vi "Scan and Trace.vi"() -> ()   [LabVIEW 2020]
uses:
  Global Parameters.vi
  <vilib>/Utility/file.llb/Write Delimited Spreadsheet (DBL).vi
panel:
  out "x-y":u32
  out "Laser On":bool
  in  "set trace data save rate(ms)":u32
  out "Current Position":dbl[](array[numeric])
  in  "stop":bool
  in  "Tab Control":T1(tab)
  in  "Graph path":path=path "I:/scan map test"
  out "Intensity Graph":dbl[][](graph)=[[150150.0, 0.0, 0.0, 0.0, 0.0, 0.0, 0.0, 0.0, 0.0, 0.0, 0.0, 0.0, 0.0, 0.0, 0.0, 0.0, 0.0, 0.0, 0.0, 0.0, 0.0, 0.0, 0.0, 0.0, 0.0, 0.0, 0.0, 0.0, 0.0, 0.0, 0.0], [150150.0, 0.0, 0.0, 0.0, 0.0, 0.0, 0.0, 0.0, 0.0, 0.0, 0.0, 0.0, 0.0, 0.0, 0.0, 0.0, 0.0, 0.0, 0.0, 0.0, 0.0, 0.0, 0.0, 0.0, 0.0, 0.0, 0.0, 0.0, 0.0, 0.0, 0.0], [150150.0, 0.0, 0.0, 0.0, 0.0, 0.0, 0.0, 0.0, 0.0, 0.0, 0.0, 0.0, 0.0, 0.0, 0.0, 0.0, 0.0, 0.0, 0.0, 0.0, 0.0, 0.0, 0.0, 0.0, 0.0, 0.0, 0.0, 0.0, 0.0, 0.0, 0.0], [150150.0, 0.0, 0.0, 0.0, 0.0, 0.0, 0.0, 0.0, 0.0, 0.0, 0.0, 0.0, 0.0, 0.0, 0.0, 0.0, 0.0, 0.0, 0.0, 0.0, 0.0, 0.0, 0.0, 0.0, 0.0, 0.0, 0.0, 0.0, 0.0, 0.0, 0.0], [150150.0, 0.0, 0.0, 0.0, 0.0, 0.0, 0.0, 0.0, 0.0, 0.0, 0.0, 0.0, 0.0, 0.0, 0.0, 0.0, 0.0, 0.0, 0.0, 0.0, 0.0, 0.0, 0.0, 0.0, 0.0, 0.0, 0.0, 0.0, 0.0, 0.0, 0.0], [150150.0, 0.0, 0.0, 0.0, 0.0, 0.0, 0.0, 0.0, 0.0, 0.0, 0.0, 0.0, 0.0, 0.0, 0.0, 0.0, 0.0, 0.0, 0.0, 0.0, 0.0, 0.0, 0.0, 0.0, 0.0, 0.0, 0.0, 0.0, 0.0, 0.0, 0.0], [150150.0, 0.0, 0.0, 0.0, 0.0, 0.0, 0.0, 0.0, 0.0, 0.0, 0.0, 0.0, 0.0, 0.0, 0.0, 0.0, 0.0, 0.0, 0.0, 0.0, 0.0, 0.0, 0.0, 0.0, 0.0, 0.0, 0.0, 0.0, 0.0, 0.0, 0.0], [150150.0, 0.0, 0.0, 0.0, 0.0, 0.0, 0.0, 0.0, 0.0, 0.0, 0.0, 0.0, 0.0, 0.0, 0.0, 0.0, 0.0, 0.0, 0.0, 0.0, 0.0, 0.0, 0.0, 0.0, 0.0, 0.0, 0.0, 0.0, 0.0, 0.0, 0.0], [150150.0, 0.0, 0.0, 0.0, 0.0, 0.0, 0.0, 0.0, 0.0, 0.0, 0.0, 0.0, 0.0, 0.0, 0.0, 0.0, 0.0, 0.0, 0.0, 0.0, 0.0, 0.0, 0.0, 0.0, 0.0, 0.0, 0.0, 0.0, 0.0, 0.0, 0.0], [150150.0, 0.0, 0.0, 0.0, 0.0, 0.0, 0.0, 0.0, 0.0, 0.0, 0.0, 0.0, 0.0, 0.0, 0.0, 0.0, 0.0, 0.0, 0.0, 0.0, 0.0, 0.0, 0.0, 0.0, 0.0, 0.0, 0.0, 0.0, 0.0, 0.0, 0.0], [150150.0, 0.0, 0.0, 0.0, 0.0, 0.0, 0.0, 0.0, 0.0, 0.0, 0.0, 0.0, 0.0, 0.0, 0.0, 0.0, 0.0, 0.0, 0.0, 0.0, 0.0, 0.0, 0.0, 0.0, 0.0, 0.0, 0.0, 0.0, 0.0, 0.0, 0.0], [150150.0, 0.0, 0.0, 0.0, 0.0, 0.0, 0.0, 0.0, 0.0, 0.0, 0.0, 0.0, 0.0, 0.0, 0.0, 0.0, 0.0, 0.0, 0.0, 0.0, 0.0, 0.0, 0.0, 0.0, 0.0, 0.0, 0.0, 0.0, 0.0, 0.0, 0.0], [150150.0, 0.0, 0.0, 0.0, 0.0, 0.0, 0.0, 0.0, 0.0, 0.0, 0.0, 0.0, 0.0, 0.0, 0.0, 0.0, 0.0, 0.0, 0.0, 0.0, 0.0, 0.0, 0.0, 0.0, 0.0, 0.0, 0.0, 0.0, 0.0, 0.0, 0.0], [150150.0, 0.0, 0.0, 0.0, 0.0, 0.0, 0.0, 0.0, 0.0, 0.0, 0.0, 0.0, 0.0, 0.0, 0.0, 0.0, 0.0, 0.0, 0.0, 0.0, 0.0, 0.0, 0.0, 0.0, 0.0, 0.0, 0.0, 0.0, 0.0, 0.0, 0.0], [150150.0, 0.0, 0.0, 0.0, 0.0, 0.0, 0.0, 0.0, 0.0, 0.0, 0.0, 0.0, 0.0, 0.0, 0.0, 0.0, 0.0, 0.0, 0.0, 0.0, 0.0, 0.0, 0.0, 0.0, 0.0, 0.0, 0.0, 0.0, 0.0, 0.0, 0.0], [0.0, 0.0, 0.0, 0.0, 0.0, 0.0, 0.0, 0.0, 0.0, 0.0, 0.0, 0.0, 0.0, 0.0, 0.0, 0.0, 0.0, 0.0, 0.0, 0.0, 0.0, 0.0, 0.0, 0.0, 0.0, 0.0, 0.0, 0.0, 0.0, 0.0, 0.0], [0.0, 0.0, 0.0, 0.0, 0.0, 0.0, 0.0, 0.0, 0.0, 0.0, 0.0, 0.0, 0.0, 0.0, 0.0, 0.0, 0.0, 0.0, 0.0, 0.0, 0.0, 0.0, 0.0, 0.0, 0.0, 0.0, 0.0, 0.0, 0.0, 0.0, 0.0], [0.0, 0.0, 0.0, 0.0, 0.0, 0.0, 0.0, 0.0, 0.0, 0.0, 0.0, 0.0, 0.0, 0.0, 0.0, 0.0, 0.0, 0.0, 0.0, 0.0, 0.0, 0.0, 0.0, 0.0, 0.0, 0.0, 0.0, 0.0, 0.0, 0.0, 0.0], [0.0, 0.0, 0.0, 0.0, 0.0, 0.0, 0.0, 0.0, 0.0, 0.0, 0.0, 0.0, 0.0, 0.0, 0.0, 0.0, 0.0, 0.0, 0.0, 0.0, 0.0, 0.0, 0.0, 0.0, 0.0, 0.0, 0.0, 0.0, 0.0, 0.0, 0.0], [0.0, 0.0, 0.0, 0.0, 0.0, 0.0, 0.0, 0.0, 0.0, 0.0, 0.0, 0.0, 0.0, 0.0, 0.0, 0.0, 0.0, 0.0, 0.0, 0.0, 0.0, 0.0, 0.0, 0.0, 0.0, 0.0, 0.0, 0.0, 0.0, 0.0, 0.0], [0.0, 0.0, 0.0, 0.0, 0.0, 0.0, 0.0, 0.0, 0.0, 0.0, 0.0, 0.0, 0.0, 0.0, 0.0, 0.0, 0.0, 0.0, 0.0, 0.0, 0.0, 0.0, 0.0, 0.0, 0.0, 0.0, 0.0, 0.0, 0.0, 0.0, 0.0], [0.0, 0.0, 0.0, 0.0, 0.0, 0.0, 0.0, 0.0, 0.0, 0.0, 0.0, 0.0, 0.0, 0.0, 0.0, 0.0, 0.0, 0.0, 0.0, 0.0, 0.0, 0.0, 0.0, 0.0, 0.0, 0.0, 0.0, 0.0, 0.0, 0.0, 0.0], [0.0, 0.0, 0.0, 0.0, 0.0, 0.0, 0.0, 0.0, 0.0, 0.0, 0.0, 0.0, 0.0, 0.0, 0.0, 0.0, 0.0, 0.0, 0.0, 0.0, 0.0, 0.0, 0.0, 0.0, 0.0, 0.0, 0.0, 0.0, 0.0, 0.0, 0.0], [0.0, 0.0, 0.0, 0.0, 0.0, 0.0, 0.0, 0.0, 0.0, 0.0, 0.0, 0.0, 0.0, 0.0, 0.0, 0.0, 0.0, 0.0, 0.0, 0.0, 0.0, 0.0, 0.0, 0.0, 0.0, 0.0, 0.0, 0.0, 0.0, 0.0, 0.0], [0.0, 0.0, 0.0, 0.0, 0.0, 0.0, 0.0, 0.0, 0.0, 0.0, 0.0, 0.0, 0.0, 0.0, 0.0, 0.0, 0.0, 0.0, 0.0, 0.0, 0.0, 0.0, 0.0, 0.0, 0.0, 0.0, 0.0, 0.0, 0.0, 0.0, 0.0], [0.0, 0.0, 0.0, 0.0, 0.0, 0.0, 0.0, 0.0, 0.0, 0.0, 0.0, 0.0, 0.0, 0.0, 0.0, 0.0, 0.0, 0.0, 0.0, 0.0, 0.0, 0.0, 0.0, 0.0, 0.0, 0.0, 0.0, 0.0, 0.0, 0.0, 0.0], [0.0, 0.0, 0.0, 0.0, 0.0, 0.0, 0.0, 0.0, 0.0, 0.0, 0.0, 0.0, 0.0, 0.0, 0.0, 0.0, 0.0, 0.0, 0.0, 0.0, 0.0, 0.0, 0.0, 0.0, 0.0, 0.0, 0.0, 0.0, 0.0, 0.0, 0.0], [0.0, 0.0, 0.0, 0.0, 0.0, 0.0, 0.0, 0.0, 0.0, 0.0, 0.0, 0.0, 0.0, 0.0, 0.0, 0.0, 0.0, 0.0, 0.0, 0.0, 0.0, 0.0, 0.0, 0.0, 0.0, 0.0, 0.0, 0.0, 0.0, 0.0, 0.0], [0.0, 0.0, 0.0, 0.0, 0.0, 0.0, 0.0, 0.0, 0.0, 0.0, 0.0, 0.0, 0.0, 0.0, 0.0, 0.0, 0.0, 0.0, 0.0, 0.0, 0.0, 0.0, 0.0, 0.0, 0.0, 0.0, 0.0, 0.0, 0.0, 0.0, 0.0], [0.0, 0.0, 0.0, 0.0, 0.0, 0.0, 0.0, 0.0, 0.0, 0.0, 0.0, 0.0, 0.0, 0.0, 0.0, 0.0, 0.0, 0.0, 0.0, 0.0, 0.0, 0.0, 0.0, 0.0, 0.0, 0.0, 0.0, 0.0, 0.0, 0.0, 0.0], [0.0, 0.0, 0.0, 0.0, 0.0, 0.0, 0.0, 0.0, 0.0, 0.0, 0.0, 0.0, 0.0, 0.0, 0.0, 0.0, 0.0, 0.0, 0.0, 0.0, 0.0, 0.0, 0.0, 0.0, 0.0, 0.0, 0.0, 0.0, 0.0, 0.0, 0.0]]
  in  "go to crusor":bool caption="X"
  in  "vertical num":u32=30
  in  "horizontal num":u32=30
  in  "horizontal range":dbl=5.0
  in  "horizontal start":dbl=5.0
  in  "vertical range":dbl=5.0
  in  "vertical start":dbl=5.0
  in  "Horizontal axis":i8(ring) items=["x", "y", "z", ""]
  in  "Vertical axis":i8(ring) items=["x", "y", "z", ""]
  out "vertical step":dbl
  out "horizontal step":dbl
  in  "Stop scan":bool
  out "counts/s":dbl format="%#.10g"
  out "H goal position":dbl[](array[numeric])
  out "V goal position":dbl[](array[numeric])
  out "Loop  indicator":i32
  out "Waveform Chart":dbl(graph)
  in  "Start moving":bool
  in  "Save trace data?":bool
  in  "-0.05 2":bool caption="X"
  in  "Tracing axis":enum16{"x", "y", "z"}(ring)=enum."z"
  in  "-01 2":bool caption="X"
  in  "Wait time(ms)":u32=200
  in  "+01 2":bool caption="X"
  in  "+0.05 2":bool caption="X"
  in  "-0.01 2":bool caption="X"
  in  "+0.01 2":bool caption="X"
  in  "Exit Tracing":bool
  out "counts rate":dbl format="%#.10g"
  in  "Trace data file path 2":path=path "trace data"
  out "Actual Duty Cycle":dbl=0.5
  out "Actual Frequency":dbl=50.0
  out "Duty Cycle":dbl=0.5 format="%.6f"
  out "Frequency":dbl=50.0 format="%.6f"
  out "Output Terminal":tag="/Dev1/PFI2"
  out "Counter":tag="Dev1/ctr0"
  out "Clock on":bool
  out "ASG连接状态":bool
  out "ASG error":errorcluster
  out "Scanner\n error":errorcluster
  in  "start":bool
  in  "Select Process Before Start":enum16{"Goto cursor", "Trace", "Scan"}(ring)
  out "Scanning":bool=TRUE
  out "Tracing":bool=TRUE
  out "Goto cursor":bool=TRUE
  # "Only for showing Clock Settings, Please go to Global Parameter to Change the Settings"
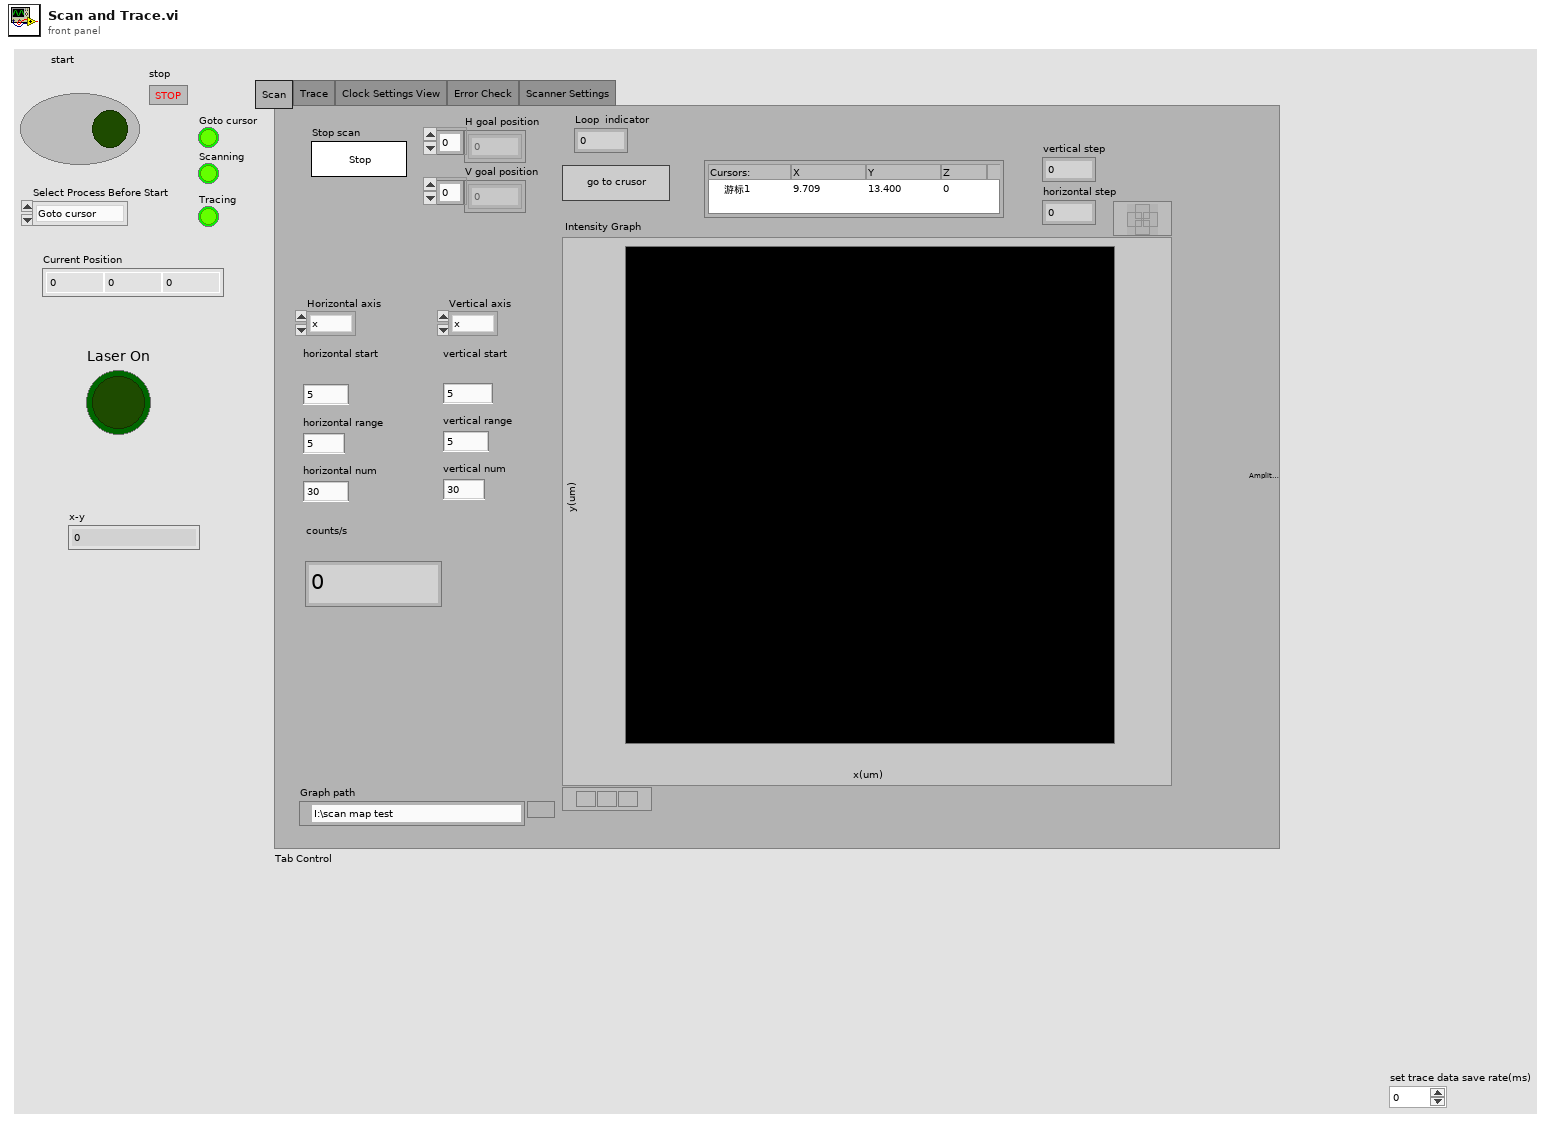
[diagram p1: front panel]
types:
  T1 = enum32{"Scan", "Trace", "Clock Settings View", "Error Check", "Scanner Settings"}
  T2 = typedef "imagedata.ctl" = cluster{"image type":i32, "image depth":i32, "image":u8[], "mask":u8[], "colors":u32[], "Rectangle":cluster{"left":i16, "top":i16, "right":i16, "bottom":i16}}
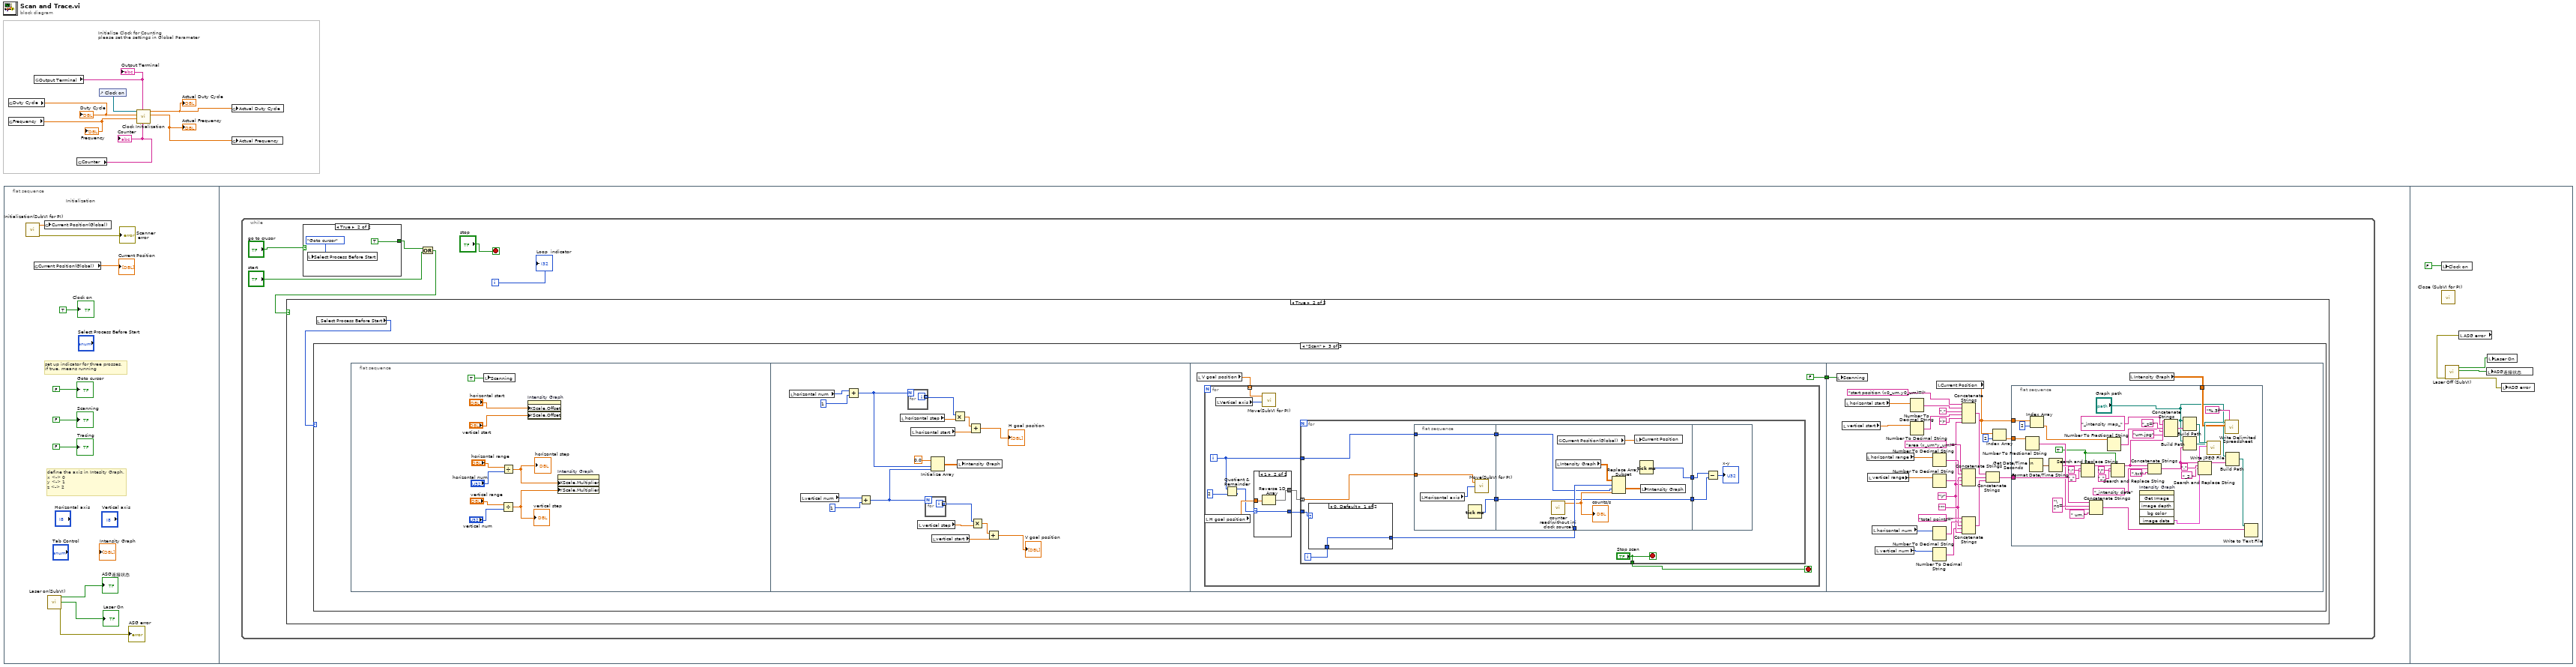
[diagram p0: block diagram]
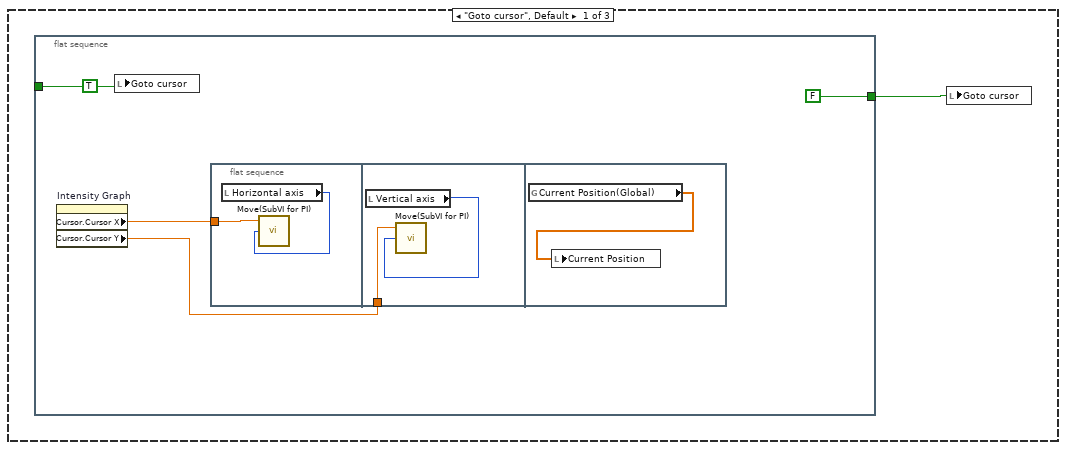
[diagram p3: hidden frame]
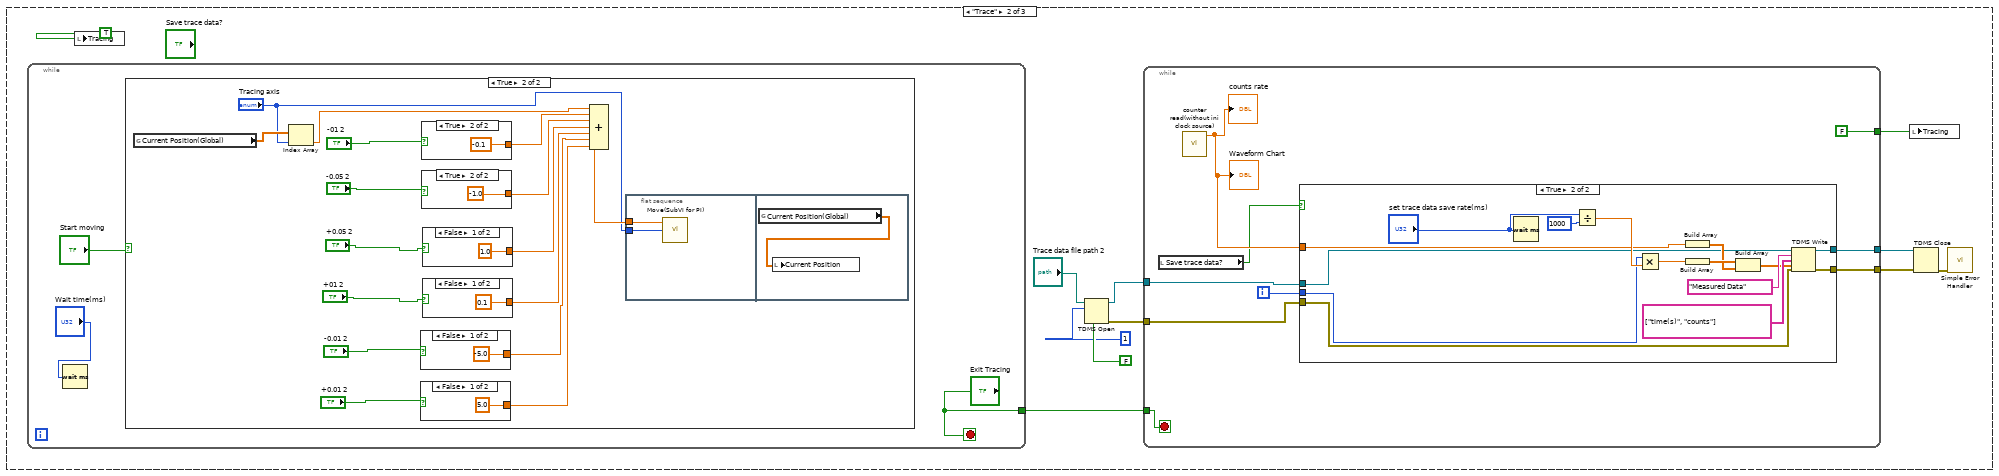
[diagram p4: hidden frame]
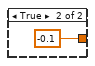
[diagram p7: hidden frame]
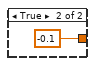
[diagram p8: hidden frame]
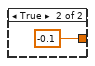
[diagram p9: hidden frame]
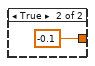
[diagram p10: hidden frame]
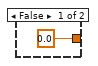
[diagram p11: hidden frame]
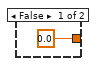
[diagram p12: hidden frame]
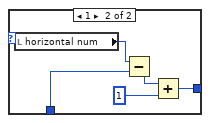
[diagram p13: hidden frame]
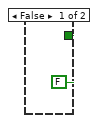
[diagram p15: hidden frame]
diagram:
  # "Initialize Clock for Counting\nplease set the settings in Global Parameter"
  n1 = flat-sequence {
    frame #0 {
      # "Initialization"
      # "define the axis in Intesity Graph,\nx <-> 0\ny <-> 1\nz <-> 2"
      # "set up indicator for three prosses,\nif true, means running"
      n2 = call "Initialization(SubVI for PI).vi"() -> ("error out"=→"Scanner\n error":errorcluster, "Position"=w12:dbl[])  [unwired: 10 in]
      n3 = global read "Global Parameters.vi" "Current Position(Global)"() -> (→"Current Position":dbl[])
      n4 = global write "Global Parameters.vi" "Current Position(Global)"(w12) -> ()
      n5 = call "Laser on(SubVI).vi"() -> ("error out"=→"ASG error":errorcluster, "Laser On"=→"Laser On":bool, "ASG Connection On?"=→"ASG连接状态":bool)  [unwired: 9 in]
      "Goto cursor" <- FALSE
      "Tracing" <- FALSE
      "Scanning" <- FALSE
      "Clock on" <- TRUE
    }
    frame #1 {
      n6 = while {
        i -> [w21]
        stop <- "stop" stop-if-true
        n7 = case shown="True" "go to crusor" {
          tunnel: [FALSE TRUE] -> w19
          frame False {
          }
          frame True {
            n8 = local write "Select Process Before Start"(enum16{"Goto cursor", "Trace", "Scan"}."Goto cursor" ("Select Process Before Start")) -> ()
          }
        }
        n9 = Or(x=w19, y="start") -> (x .or. y?=w18:bool)
        n10 = case shown="True" w18 {
          frame False {
          }
          frame True {
            n11 = local read "Select Process Before Start"() -> (w24:enum16{"Goto cursor", "Trace", "Scan"})
            n12 = case shown="\"Scan\"" w24 {
              frame "Goto cursor", Default {
                n13 = flat-sequence {
                  tunnel: TRUE -> [w28]
                  tunnel: [FALSE] -> w25
                  frame #0 {
                    n14 = property on="Intensity Graph" class="IntGraph (strict)"() -> ("Cursor.Cursor X"=w30:dbl, "Cursor.Cursor Y"=w29:dbl)  [unwired: 2 in, 2 out]
                    n15 = local write "Goto cursor"(w28) -> ()
                    n16 = flat-sequence {
                      tunnel: w30 -> [w32]
                      tunnel: w29 -> [w34]
                      frame #0 {
                        n17 = local read "Horizontal axis"() -> (w31:i8)
                        n18 = call "Move(SubVI for PI).vi"("Numeric"=w32, "index"=w31) -> ()  [unwired: 5 in, 1 out]
                      }
                      frame #1 {
                        n19 = local read "Vertical axis"() -> (w33:i8)
                        n20 = call "Move(SubVI for PI).vi"("Numeric"=w34, "index"=w33) -> ()  [unwired: 5 in, 1 out]
                      }
                      frame #2 {
                        n21 = global read "Global Parameters.vi" "Current Position(Global)"() -> (w35:dbl[])
                        n22 = local write "Current Position"(w35) -> ()
                      }
                    }
                  }
                }
                n23 = local write "Goto cursor"(w25) -> ()
              }
              frame "Trace" {
                n24 = while {
                  tunnel: ["Exit Tracing"] -> w44
                  stop <- "Exit Tracing" stop-if-true
                  n25 = Wait (ms)(milliseconds to wait="Wait time(ms)") -> ()  [unwired: 1 out]
                  n26 = case shown="True" "Start moving" {
                    frame False {
                    }
                    frame True {
                      n27 = global read "Global Parameters.vi" "Current Position(Global)"() -> (w91:dbl[])
                      n28 = Index Array(array=w91, index="Tracing axis") -> (element=w84:dbl)
                      n29 = case shown="False" "-0.01 2" {
                        tunnel: [-5.0 -0.1] -> w86
                        frame False {
                        }
                        frame True {
                        }
                      }
                      n30 = case shown="False" "+0.01 2" {
                        tunnel: [5.0 -0.1] -> w85
                        frame False {
                        }
                        frame True {
                        }
                      }
                      n31 = case shown="True" "-01 2" {
                        tunnel: [0.0 -0.1] -> w90
                        frame False {
                        }
                        frame True {
                        }
                      }
                      n32 = case shown="True" "-0.05 2" {
                        tunnel: [0.0 -1.0] -> w89
                        frame False {
                        }
                        frame True {
                        }
                      }
                      n33 = case shown="False" "+0.05 2" {
                        tunnel: [1.0 -0.1] -> w88
                        frame False {
                        }
                        frame True {
                        }
                      }
                      n34 = case shown="False" "+01 2" {
                        tunnel: [0.1 -0.1] -> w87
                        frame False {
                        }
                        frame True {
                        }
                      }
                      n35 = Compound Arithmetic op=ADD(w84, w90, w89, w88, w87, w86, w85) -> (w77:dbl)
                      n36 = flat-sequence {
                        tunnel: w77 -> [w105]
                        tunnel: "Tracing axis" -> [w104]
                        frame #0 {
                          n37 = call "Move(SubVI for PI).vi"("Numeric"=w105, "index"=w104) -> ()  [unwired: 5 in, 1 out]
                        }
                        frame #1 {
                          n38 = global read "Global Parameters.vi" "Current Position(Global)"() -> (w106:dbl[])
                          n39 = local write "Current Position"(w106) -> ()
                        }
                      }
                    }
                  }
                }
                n40 = local write "Tracing"(TRUE) -> ()
                n41 = TDMS Open(6:FALSE ("disable buffering (T)"), 10:1, 11:"Trace data file path 2") -> (0:w43:errorcluster, 3:w42:refnum<k34>)  [unwired: 4 in]
                n42 = while {
                  tunnel: w44 -> [w55]
                  tunnel: w43 -> [w53]
                  tunnel: w42 -> [w52]
                  tunnel: [w49] -> w40
                  tunnel: [w48] -> w39
                  tunnel: [FALSE] -> w38
                  i -> [w54]
                  stop <- w55 stop-if-true
                  n43 = local read "Save trace data?"() -> (w50:bool)
                  n44 = call "counter read(without ini clock source).vi"() -> ("counter rate"=w51:dbl)  [unwired: 11 in]
                  "counts rate" <- w51
                  "Waveform Chart" <- w51
                  n45 = case shown="True" w50 {
                    tunnel: w52 -> [w57 w64]
                    tunnel: [w57 w63] -> w49
                    tunnel: w51 -> [_ w62]
                    tunnel: w53 -> [w56 w61]
                    tunnel: [w56 w60] -> w48
                    tunnel: w54 -> [_ w59]
                    frame False {
                    }
                    frame True {
                      n46 = Wait (ms)(milliseconds to wait="set trace data save rate(ms)") -> ()  [unwired: 1 out]
                      n47 = Divide(x="set trace data save rate(ms)", y=u32 1000) -> (x/y=w66:dbl)
                      n48 = Multiply(x=w59, y=w66) -> (x*y=w65:dbl)
                      n49 = Build Array(w62) -> (w69:dbl[])
                      n50 = Build Array(w65) -> (w70:dbl[])
                      n51 = Build Array(w70, w69) -> (w68:dbl[][])
                      n52 = TDMS Write(0:w64, 5:"Measured Data" ("group name"), 7:string[] ["time(s)", "counts"] ("channel names"), 9:w68, 11:w61) -> (4:w63:refnum<k34>, 15:w60:errorcluster)  [unwired: 1 in, 2 out]
                    }
                  }
                }
                n53 = local write "Tracing"(w38) -> ()
                n54 = TDMS Close(8:w39, 11:w40) -> (0:w41:errorcluster)  [unwired: 1 out]
                n55 = call <vilib>:"Simple Error Handler.vi"("error in (no error)"=w41) -> ()  [unwired: 1 in, 8 out]
              }
              frame "Scan" {
                n56 = flat-sequence {
                  tunnel: [FALSE] -> w107
                  tunnel: w107 -> [w211]
                  frame #0 {
                    n57 = local write "Scanning"(TRUE) -> ()
                    n58 = Divide(x="vertical range", y="vertical num") -> (x/y=w108:dbl)
                    "vertical step" <- w108
                    n59 = Divide(x="horizontal range", y="horizontal num") -> (x/y=w109:dbl)
                    "horizontal step" <- w109
                    n60 = property on="Intensity Graph" class="IntGraph (strict)"("XScale.Offset"="horizontal start", "YScale.Offset"="vertical start") -> ()  [unwired: 2 in, 2 out]
                    n61 = property on="Intensity Graph" class="IntGraph (strict)"("XScale.Multiplier"=w109, "YScale.Multiplier"=w108) -> ()  [unwired: 2 in, 2 out]
                  }
                  frame #1 {
                    n62 = local read "horizontal num"() -> (w119:u32)
                    n63 = local read "vertical num"() -> (w122:u32)
                    n64 = Add(x=w119, y=1) -> (x+y=w118:u32)
                    n65 = Add(x=w122, y=1) -> (x+y=w117:u32)
                    n66 = local read "horizontal step"() -> (w133:dbl)
                    n67 = for {
                      N: w118 -> [_]
                      tunnel: [w136] -> w134 mode=indexing
                      i -> [w136]
                    }
                    n68 = local read "horizontal start"() -> (w131:dbl)
                    n69 = local read "vertical step"() -> (w128:dbl)
                    n70 = for {
                      N: w117 -> [_]
                      tunnel: [w135] -> w129 mode=indexing
                      i -> [w135]
                    }
                    n71 = Initialize Array(0.0, w118, w117) -> (w123:dbl[][])
                    n72 = local read "vertical start"() -> (w126:dbl)
                    n73 = Multiply(x=w134, y=w133) -> (x*y=w132:dbl[])
                    n74 = local write "Intensity Graph"(w123) -> ()
                    n75 = Add(x=w132, y=w131) -> (x+y=→"H goal position":dbl[])
                    n76 = Multiply(x=w129, y=w128) -> (x*y=w127:dbl[])
                    n77 = Add(x=w127, y=w126) -> (x+y=→"V goal position":dbl[])
                  }
                  frame #2 {
                    n78 = local read "V goal position"() -> (w138:dbl[])
                    n79 = for {
                      tunnel: w138 -> [w140] mode=indexing
                      i -> [w142]
                      stop <- w141 stop-if-true
                      n80 = local read "H goal position"() -> (w146:dbl[])
                      n81 = local read "Vertical axis"() -> (w139:i8)
                      n82 = Quotient & Remainder(x=w142, y=2) -> (x-y*floor(x/y)=w145:i32)  [unwired: 1 out]
                      n83 = case shown="1" w145 {
                        selector: w145 -> [w179 w181]
                        tunnel: w146 -> [w180 w183]
                        tunnel: [w180 w182] -> w144
                        tunnel: [w179 w181] -> w143
                        frame 0, Default {
                        }
                        frame 1 {
                          n84 = Reverse 1D Array(array=w183) -> (reversed array=w182:dbl[])
                        }
                      }
                      n85 = call "Move(SubVI for PI).vi"("Numeric"=w140, "index"=w139) -> ()  [unwired: 5 in, 1 out]
                      n86 = for {
                        tunnel: w144 -> [w157] mode=indexing
                        tunnel: w143 -> [w156]
                        tunnel: w142 -> [w153]
                        tunnel: ["Stop scan"] -> w141
                        i -> [w155]
                        stop <- "Stop scan" stop-if-true
                        n87 = case shown="0, Default" w156 {
                          tunnel: w155 -> [w158 w162]
                          tunnel: [w158 w159] -> w154
                          frame 0, Default {
                          }
                          frame 1 {
                            n88 = local read "horizontal num"() -> (w163:u32)
                            n89 = Subtract(x=w163, y=w162) -> (x-y=w161:u32)
                            n90 = Add(x=w161, y=1) -> (x+y=w159:u32)
                          }
                        }
                        n91 = flat-sequence {
                          tunnel: w157 -> [w166]
                          tunnel: w153 -> [w167]
                          tunnel: [w167] -> w151
                          tunnel: [w164] -> w149
                          tunnel: w154 -> [w174]
                          tunnel: w151 -> [w173]
                          tunnel: [w169] -> w150
                          tunnel: w149 -> [w169]
                          tunnel: [w168] -> w148
                          tunnel: w150 -> [w176]
                          tunnel: w148 -> [w177]
                          frame #0 {
                            n92 = local read "Horizontal axis"() -> (w165:i8)
                            n93 = Tick Count (ms)() -> (millisecond timer value=w164:u32)
                            n94 = call "Move(SubVI for PI).vi"("Numeric"=w166, "index"=w165) -> ()  [unwired: 5 in, 1 out]
                          }
                          frame #1 {
                            n95 = call "counter read(without ini clock source).vi"() -> ("counter rate"=w172:dbl)  [unwired: 11 in]
                            "counts/s" <- w172
                            n96 = local read "Intensity Graph"() -> (w175:dbl[][])
                            n97 = global read "Global Parameters.vi" "Current Position(Global)"() -> (w170:dbl[])
                            n98 = Replace Array Subset(array=w175, new element=w172, index (row)=w174, index (col)=w173) -> (w171:dbl[][])
                            n99 = local write "Current Position"(w170) -> ()
                            n100 = Tick Count (ms)() -> (millisecond timer value=w168:u32)
                            n101 = local write "Intensity Graph"(w171) -> ()
                          }
                          frame #2 {
                            n102 = Subtract(x=w177, y=w176) -> (x-y=→"x-y":u32)
                          }
                        }
                      }
                    }
                  }
                  frame #3 {
                    w200 = "\r"
                    w202 = "*" ("string")
                    n103 = local write "Scanning"(w211) -> ()
                    n104 = local read "vertical start"() -> (w191:dbl)
                    n105 = local read "horizontal start"() -> (w192:dbl)
                    n106 = local read "horizontal range"() -> (w189:dbl)
                    n107 = local read "vertical range"() -> (w188:dbl)
                    n108 = local read "horizontal num"() -> (w195:u32)
                    n109 = local read "vertical num"() -> (w194:u32)
                    n110 = Number To Decimal String(number=w192) -> (decimal integer string=w209:string)  [unwired: 1 out]
                    n111 = Number To Decimal String(number=w191) -> (decimal integer string=w207:string)  [unwired: 1 out]
                    n112 = Number To Decimal String(number=w189) -> (decimal integer string=w204:string)  [unwired: 1 out]
                    n113 = Number To Decimal String(number=w188) -> (decimal integer string=w190:string)  [unwired: 1 out]
                    n114 = Number To Decimal String(number=w195) -> (decimal integer string=w201:string)  [unwired: 1 out]
                    n115 = Number To Decimal String(number=w194) -> (decimal integer string=w193:string)  [unwired: 1 out]
                    n116 = local read "Current Position"() -> (w184:dbl[])
                    n117 = Concatenate Strings("start position (x0_um,y0_um)=(" ("string"), w209, "," ("string"), w207, ")" ("string"), w200) -> (w199:string)
                    n118 = Concatenate Strings("area (x_um*y_um)=" ("string"), w204, w202, w190, w200) -> (w198:string)
                    n119 = Concatenate Strings("total points=" ("string"), w201, w202, w193, w200) -> (w197:string)
                    n120 = Concatenate Strings(w199, w198, w197) -> (w196:string)
                    n121 = Index Array(array=w184, index=2) -> (element=w186:dbl)
                    n122 = flat-sequence {
                      tunnel: w185 -> [w214]
                      tunnel: w196 -> [w227]
                      tunnel: w186 -> [w225]
                      tunnel: w184 -> [w220]
                      frame #0 {
                        w217 = TRUE ("replace all? (F)")
                        n123 = Number To Fractional String(number=w225) -> (F-format string=w224:string)  [unwired: 3 in]
                        n124 = Get Date/Time In Seconds() -> (seconds since 1Jan1904=w247:timestamp)
                        n125 = Index Array(array=w220, index=2 ("索引")) -> (element=w218:dbl)
                        n126 = Format Date/Time String(seconds (now)=w247) -> (date/time string=w241:string)  [unwired: 2 out]
                        n127 = Search and Replace String(replace all?=w217, input string=w241, search string=":", replace string="_" ("replace string (\"\")")) -> (result string=w244:string)  [unwired: 1 in, 6 out]
                        n128 = Concatenate Strings(w227, "\nz=" ("字符串"), w224, " um." ("字符串")) -> (w226:string)
                        n129 = Number To Fractional String(number=w218) -> (F-format string=w221:string)  [unwired: 3 in]
                        n130 = Search and Replace String(replace all?=w217, input string=w244, search string="/", replace string="_" ("replace string (\"\")")) -> (result string=w232:string)  [unwired: 1 in, 6 out]
                        n131 = invoke on="Intensity Graph" class="IntGraph (strict)" method="Get Image"() -> ("image data"=w213:T2)  [unwired: 6 in, 5 out]
                        n132 = Concatenate Strings(w232, "_intensity date" ("string"), ".txt" ("string")) -> (w237:string)
                        n133 = Concatenate Strings(w232, "_intensity map_" ("string"), "_z=" ("字符串"), w221, "um.jpg" ("string")) -> (w240:string)
                        n134 = Build Path(base path="Graph path", name or relative path=w240) -> (appended path=w239:path)
                        n135 = Build Path(base path="Graph path", name or relative path=w237) -> (appended path=w215:path)
                        n136 = Search and Replace String(input string=w237, search string="." ("substring (\"\")"), replace string="_2." ("replace string (\"\")")) -> (result string=w234:string)  [unwired: 1 in, 7 out]
                        n137 = call <vilib>:"Write JPEG File.vi"("image data"=w213, "path to JPEG file"=w239) -> ()  [unwired: 1 in, 9 out]
                        n138 = call-poly <vilib>:"Write Delimited Spreadsheet.vi"("file path (dialog if empty)"=w215, "format (%.3f)"="%.3f", "2D data"=w214) -> ()  [unwired: 11 in, 2 out]
                        n139 = Build Path(base path="Graph path", name or relative path=w234) -> (appended path=w233:path)
                        n140 = Write to Text File(file (use dialog)=w233, text=w226) -> ()  [unwired: 1 in, 4 out]
                      }
                    }
                    n141 = local read "Intensity Graph"() -> (w185:dbl[][])
                  }
                }
              }
            }
          }
        }
        "Loop  indicator" <- w21
      }
    }
    frame #2 {
      n142 = local write "Clock on"(FALSE) -> ()
      n143 = call "Close (SubVI for PI).vi"() -> ()  [unwired: 12 in]
      n144 = local read "ASG error"() -> (w251:errorcluster)
      n145 = call "Laser Off (SubVI).vi"("error in (no error)"=w251) -> ("error out"=w252:errorcluster, "ASG Connection on"=w253:bool, "Laser On"=w254:bool)  [unwired: 8 in]
      n146 = local write "ASG连接状态"(w253) -> ()
      n147 = local write "Laser On"(w254) -> ()
      n148 = local write "ASG error"(w252) -> ()
    }
  }
  n149 = global read "Global Parameters.vi" "Duty Cycle"() -> (w4:dbl)
  "Duty Cycle" <- w4
  n150 = global read "Global Parameters.vi" "Frequency"() -> (w3:dbl)
  "Frequency" <- w3
  n151 = global read "Global Parameters.vi" "Output Terminal"() -> (w5:tag)
  "Output Terminal" <- w5
  n152 = global read "Global Parameters.vi" "Counter"() -> (w6:tag)
  "Counter" <- w6
  n153 = control-ref of="Clock on"() -> (w7:refnum<vi>)
  n154 = call "Clock Initialization.vi"("Counter"=w6, "Output Terminal"=w5, "Frequency"=w3, "Duty Cycle"=w4, "Boolean in"=w7) -> ("Actual Frequency"=w1:dbl, "Actual Duty Cycle"=w2:dbl)  [unwired: 5 in]
  "Actual Duty Cycle" <- w2
  "Actual Frequency" <- w1
  n155 = global write "Global Parameters.vi" "Actual Duty Cycle"(w2) -> ()
  n156 = global write "Global Parameters.vi" "Actual Frequency"(w1) -> ()
